vi "ActorRefContainer Read Logs.vi"(8 "error in (no error)":errorcluster, 11 "ActorRefContainer in":refnum<class "ActorRefContainer.lvclass">) -> (0 "error out":errorcluster, 2 "Logs":T1, 3 "ActorRefContainer out":refnum<class "ActorRefContainer.lvclass">)   [LabVIEW 2019, in "ActorRefContainer.lvlib" / "ActorRefContainer.lvclass"]
uses:
  ActorRefContainer.lvclass
  <vilib>/ActorFramework/Message Enqueuer/Message Enqueuer.lvclass
  ActorRefContainer.lvclass/ActorRefContainer.ctl
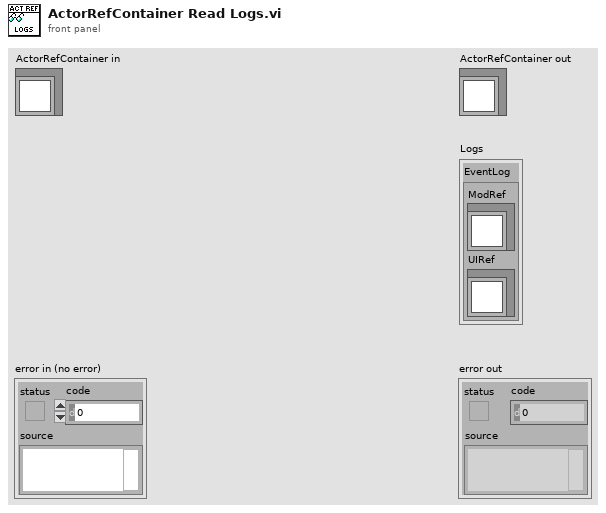
[diagram p1: front panel]
types:
  T1 = cluster{"EventLog":cluster{"ModRef":refnum<class "Message Enqueuer.lvclass">, "UIRef":refnum<class "Message Enqueuer.lvclass">}}
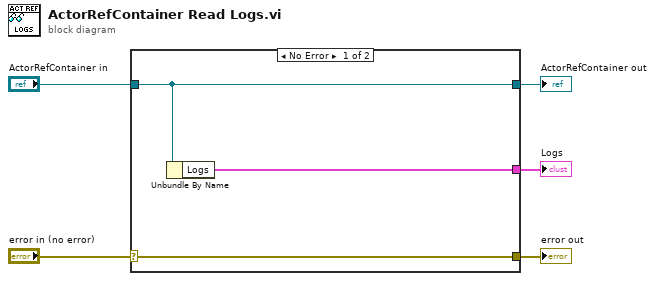
[diagram p0: block diagram]
diagram:
  n1 = case shown="No Error" "error in (no error)" {
    selector: "error in (no error)" -> [w8 w9]
    tunnel: [w8 w9] -> w4
    tunnel: [w7 w10] -> w2
    tunnel: "ActorRefContainer in" -> [w7 w10]
    tunnel: [w6 _] -> w1
    frame No Error {
      n2 = Unbundle By Name(w7) -> ("Logs"=w6:T1)
    }
    frame Error {
    }
  }
  "error out" <- w4
  "ActorRefContainer out" <- w2
  "Logs" <- w1
